vi "Parameter XML Write (ni-ballard).vi"(8 "error in":errorcluster, 10 "Parameter Array":T1[](array[typedef]), 11 "parameter file in":refnum<k24>) -> (0 "error out":errorcluster, 3 "parameter file out":refnum<k24>)   [LabVIEW 2020]
uses:
  Controls/Database_Array.ctl
  Controls/Encoding.ctl
  C:/Users/Administrator/Desktop/GIT/Ballard-Arinc-429-XML-Generator/Source/Assemblies/Ballard_Parameter_ni/bin/Debug/Parameters_Arinc429_XML_Tools.dll
  Assemblies/Ballard_Parameter_ni/bin/Debug/Parameters_Arinc429_XML_Tools.dll
  Libraries/Ballard_Parameter_ni/_tyedefs/label_type.ctl
  Libraries/Ballard_Parameter_ni/_tyedefs/parameter_type.ctl
  <userlib>/_OpenG.lib/array/array.llb/Remove Duplicates from 1D Array (I32)__ogtk.vi
  <userlib>/_OpenG.lib/array/array.llb/Filter 1D Array with Scalar (I32)__ogtk.vi
  <userlib>/_OpenG.lib/array/array.llb/Index 1D Array Elements (Variant)__ogtk.vi
  Libraries/Ballard_Parameter_ni/Ballard_429_Parameter_ni.lvlib
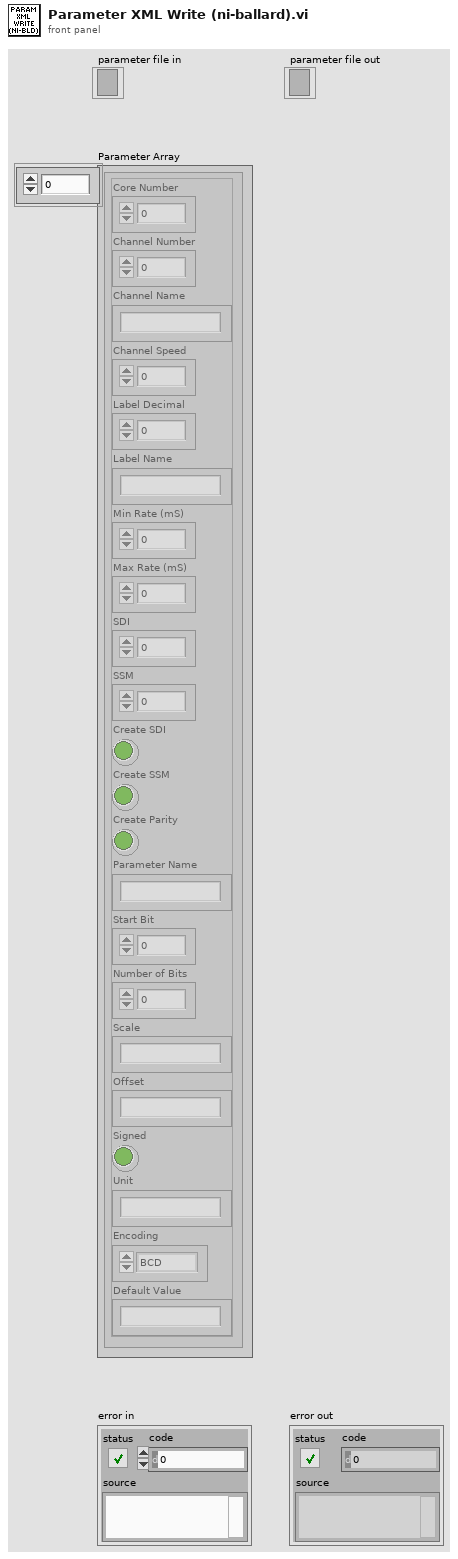
[diagram p1: front panel]
types:
  T1 = typedef "Database_Array.ctl" = cluster{"Core Number":i32, "Channel Number":i32, "Channel Name":string, "Channel Speed":i32, "Label Decimal":i32, "Label Name":string, "Min Rate (mS)":i32, "Max Rate (mS)":i32, "SDI":i32, "SSM":i32, "Create SDI":bool, "Create SSM":bool, "Create Parity":bool, "Parameter Name":string, "Start Bit":i32, "Number of Bits":i32, "Scale":string, "Offset":string, "Signed":bool, "Unit":string, "Encoding":T2, "Default Value":string}
  T2 = typedef "Encoding.ctl" = enum16{"BCD", "BNR", "Discrete"}
  T3 = typedef "Ballard_429_Parameter_ni.lvlib/label_type.ctl" = cluster{"createParityChannel":bool, "createSDIChannel":bool, "createSSMChannel":bool, "createTimestampChannel":bool, "labelDecimal":i32, "labelDecimalSpecified":bool, "labelOctal":i32, "labelOctalSpecified":bool, "sdi":i32, "transferType":i32}
  T4 = typedef "Ballard_429_Parameter_ni.lvlib/parameter_type.ctl" = cluster{"defaultValue":dbl, "encoding":i32, "name":string, "numberOfBits":i32, "offset":dbl, "scale":dbl, "signed":bool, "startBit":i32, "unit":string, "direction":i32}
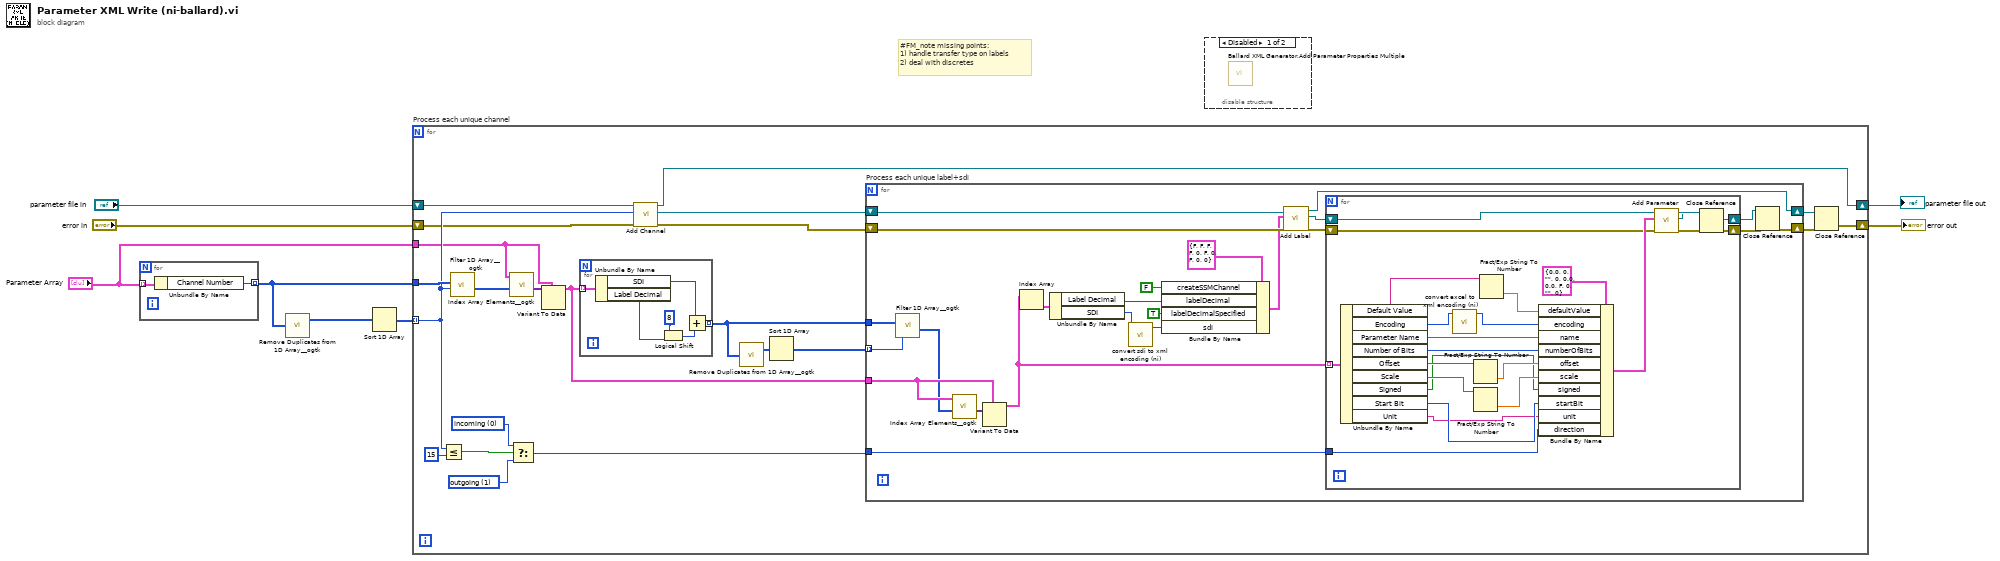
[diagram p0: block diagram]
diagram:
  # "#FM_note missing points:\n1) handle transfer type on labels\n2) deal with discretes"
  n1 = for {
    tunnel: [w10] -> w5 mode=indexing
    tunnel: "Parameter Array" -> [w9] mode=indexing
    n2 = Unbundle By Name(w9) -> ("Channel Number"=w10:i32)
  }
  n3 = call-poly <userlib>:"Remove Duplicates from 1D Array__ogtk.vi"("Input Array"=w5) -> ("Output Array"=w7:i32[])  [unwired: 1 out]
  n4 = Sort 1D Array(array=w7) -> (sorted array=w8:i32[])
  n5 = for "Process each unique channel" {
    tunnel: w8 -> [w31] mode=indexing
    tunnel: w5 -> [w32]
    tunnel: "Parameter Array" -> [w29]
    shift-right: [w27] -> w2
    shift-left: "parameter file in" -> [w28]
    shift-right: [w25] -> w1
    shift-left: "error in" -> [w26]
    w13 = 1 items=["incoming", "outgoing"] ("direction")
    w12 = 0 items=["incoming", "outgoing"] ("direction")
    n6 = Less Or Equal?(x=w31, y=15) -> (x <= y?=w14:bool)
    n7 = call-poly <userlib>:"Filter 1D Array__ogtk.vi"("items to filter"=w31, "array"=w32) -> ("filtered item indices"=w21:i32[])  [unwired: 4 in, 1 out]
    n8 = call-poly <userlib>:"Index Array Elements__ogtk.vi"("indices"=w21, "array"=w29) -> ("elements"=w22:variant[])  [unwired: 9 in]
    n9 = Select(t=w12, s=w14, f=w13) -> (s? t:f=w11:i32)
    n10 = Variant To Data(type=w29, Variant=w22) -> (data=w20:T1[])  [unwired: 1 in, 1 out]
    n11 = for {
      tunnel: w20 -> [w38] mode=indexing
      tunnel: [w34] -> w19 mode=indexing
      n12 = Unbundle By Name(w38) -> ("SDI"=w33:i32, "Label Decimal"=w35:i32)
      n13 = Logical Shift(y=i16 8, x=w35) -> (x << y=w37:i32)
      n14 = Add(x=w33, y=w37) -> (x+y=w34:i32)
    }
    n15 = call "Add Channel.vi"("error in"=w26, "hardwareChannel"=w31, "parameter file in"=w28) -> ("error out"=w17:errorcluster, "new channel"=w18:refnum<k24>, "parameter file out"=w27:refnum<k24>)  [unwired: 6 in]
    n16 = call-poly <userlib>:"Remove Duplicates from 1D Array__ogtk.vi"("Input Array"=w19) -> ("Output Array"=w24:i32[])  [unwired: 1 out]
    n17 = Sort 1D Array(array=w24) -> (sorted array=w23:i32[])
    n18 = for "Process each unique label+sdi" {
      tunnel: w23 -> [w60] mode=indexing
      tunnel: w19 -> [w61]
      tunnel: w20 -> [w58]
      shift-right: [w56] -> w15
      shift-left: w18 -> [w57]
      shift-right: [w43] -> w16
      shift-left: w17 -> [w55]
      tunnel: w11 -> [w42]
      n19 = call-poly <userlib>:"Filter 1D Array__ogtk.vi"("items to filter"=w60, "array"=w61) -> ("filtered item indices"=w41:i32[])  [unwired: 4 in, 1 out]
      n20 = call-poly <userlib>:"Index Array Elements__ogtk.vi"("indices"=w41, "array"=w58) -> ("elements"=w59:variant[])  [unwired: 9 in]
      n21 = Variant To Data(type=w58, Variant=w59) -> (data=w46:T1[])  [unwired: 1 in, 1 out]
      n22 = Index Array(array=w46) -> (element=w52:T1)  [unwired: 1 in]
      n23 = Unbundle By Name(w52) -> ("Label Decimal"=w49:i32, "SDI"=w40:i32)
      n24 = call "convert sdi to xml encoding (ni).vi"("SDI"=w40) -> ("xml sdi format"=w39:i32)  [unwired: 10 in]
      n25 = Bundle By Name(cluster=T3 {"createParityChannel"=FALSE, "createSDIChannel"=FALSE, "createSSMChannel"=FALSE, "createTimestampChannel"=FALSE, "labelDecimal"=0, "labelDecimalSpecified"=FALSE, "labelOctal"=0, "labelOctalSpecified"=FALSE, "sdi"=0, "transferType"=0} ("label configuration"), "createSSMChannel"=FALSE, "labelDecimal"=w49, "labelDecimalSpecified"=TRUE, "sdi"=w39) -> (w53:T3)
      n26 = call "Add Label.vi"("error in"=w55, "label configuration"=w53, "channel in"=w57) -> ("error out"=w48:errorcluster, "new label"=w47:refnum<k24>, "channel out"=w56:refnum<k24>)  [unwired: 6 in]
      n27 = for {
        shift-right: [w80] -> w45
        shift-left: w48 -> [w77]
        shift-right: [w83] -> w44
        shift-left: w47 -> [w84]
        tunnel: w46 -> [w62] mode=indexing
        tunnel: w42 -> [w76]
        n28 = Unbundle By Name(w62) -> ("Default Value"=w75:string, "Encoding"=w64:T2, "Parameter Name"=w68:string, "Number of Bits"=w69:i32, "Offset"=w73:string, "Scale"=w71:string, "Signed"=w67:bool, "Start Bit"=w66:i32, "Unit"=w65:string)
        n29 = call "convert excel to xml encoding (ni).vi"("excel encoding"=w64) -> ("xml encoding"=w63:i32)  [unwired: 10 in]
        n30 = Fract/Exp String To Number(string=w73) -> (number=w72:dbl)  [unwired: 3 in, 1 out]
        n31 = Fract/Exp String To Number(string=w71) -> (number=w70:dbl)  [unwired: 3 in, 1 out]
        n32 = Fract/Exp String To Number(string=w75) -> (number=w74:dbl)  [unwired: 3 in, 1 out]
        n33 = Bundle By Name(cluster=T4 {"defaultValue"=0.0, "encoding"=0, "name"="", "numberOfBits"=0, "offset"=0.0, "scale"=0.0, "signed"=FALSE, "startBit"=0, "unit"="", "direction"=0} ("parameter configuration"), "defaultValue"=w74, "encoding"=w63, "name"=w68, "numberOfBits"=w69, "offset"=w72, "scale"=w70, "signed"=w67, "startBit"=w66, "unit"=w65, "direction"=w76) -> (w78:T4)
        n34 = call "Add Parameter.vi"("error in"=w77, "parameter configuration"=w78, "label in"=w84) -> ("error out"=w81:errorcluster, "new parameter"=w82:refnum<k24>, "label out"=w83:refnum<k24>)  [unwired: 6 in]
        n35 = Close Reference(reference=w82, error in (no error)=w81) -> (error out=w80:errorcluster)
      }
      n36 = Close Reference(reference=w44, error in (no error)=w45) -> (error out=w43:errorcluster)
    }
    n37 = Close Reference(reference=w15, error in (no error)=w16) -> (error out=w25:errorcluster)
  }
  "parameter file out" <- w2
  "error out" <- w1
  n38 = disable-structure shown="Disabled" {
    frame Disabled {
      n39 = call "Ballard XML Generator.Add Parameter Properties Multiple.vi"() -> ()  [unwired: 15 in, 1 out]
    }
    frame Enabled {
    }
  }
